vi "Init RemoteDataService.vi"(8 "error in (no error)":errorcluster, 11 "Vecto in":refnum<class "Vecto.lvclass">) -> (0 "error out":errorcluster, 3 "Vecto out":refnum<class "Vecto.lvclass">)   [LabVIEW 2020, in "Vecto.lvlib" / "Vecto.lvclass"]
uses:
  Vecto.lvclass
  Vecto.lvclass/Vecto.ctl
  RemoteDataService/RemoteDataService.lvclass
  Node Config/Node Config.lvclass
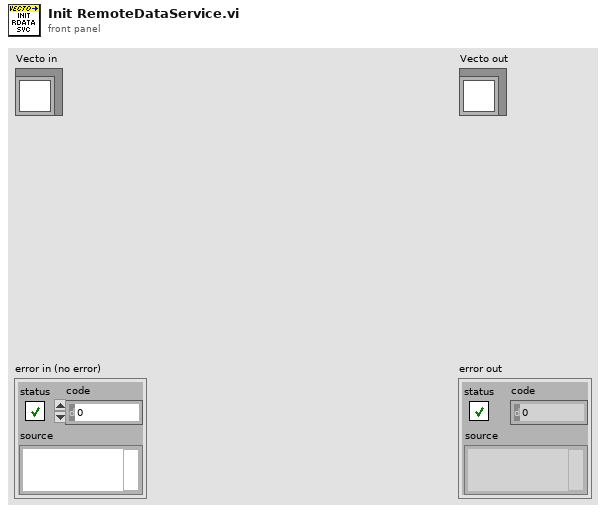
[diagram p1: front panel]
types:
  T1 = typedef "VectoConfig.lvlib/Telemetry Config.ctl" = cluster{"Routing":T2, "Endpoint":T3}
  T2 = typedef "VectoConfig.lvlib/Telemetry Routing.ctl" = enum16{"Multicast", "Unicast"}
  T3 = typedef "VectoConfig.lvlib/Endpoint.ctl" = cluster{"Address":string, "Port":u16}
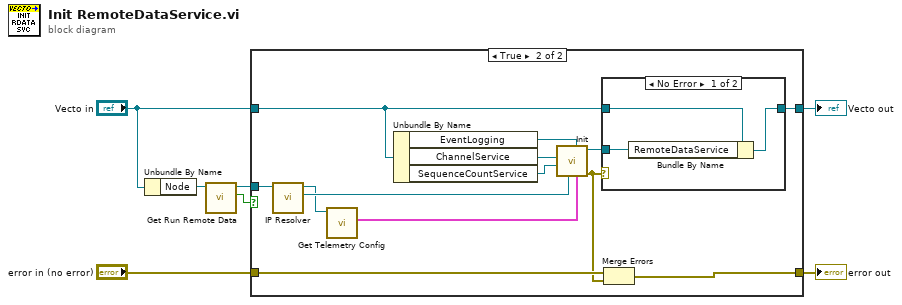
[diagram p0: block diagram]
diagram:
  n1 = Unbundle By Name("Vecto in") -> ("Node"=w5:refnum<class "Node Config.lvclass">)
  n2 = call "Get Run Remote Data.vi"("Node Config in"=w5) -> ("Run Remote Data"=w4:bool, "Node Config out"=w1:refnum<class "Node Config.lvclass">)  [unwired: 8 in, 1 out]
  n3 = case shown="True" w4 {
    tunnel: [w8 w22] -> w7
    tunnel: "Vecto in" -> [w8 w18]
    tunnel: "error in (no error)" -> [w9 w17]
    tunnel: [w9 w16] -> w2
    tunnel: w1 -> [_ w13]
    frame False {
    }
    frame True {
      n4 = call "IP Resolver.vi"("Node Config in"=w13) -> ("IP Resolver"=w12:refnum<class "IP Resolver.lvclass">, "Node Config out"=w11:refnum<class "Node Config.lvclass">)  [unwired: 8 in, 1 out]
      n5 = call "Get Telemetry Config.vi"("Node Config in"=w11) -> ("Telemtry Config"=w10:T1)  [unwired: 8 in, 2 out]
      n6 = Unbundle By Name(w18) -> ("EventLogging"=w14:refnum<class "EventLoggingService.lvclass">, "ChannelService"=w20:refnum<class "ChannelService.lvclass">, "SequenceCountService"=w19:refnum<class "SequenceCountService.lvclass">)
      n7 = call "Init.vi"("Telemtry Config (Multicast)"=w10, "EventLogger"=w14, "IP Resolver"=w12, "SequenceCountService"=w19, "ChannelService"=w20) -> ("error out"=w15:errorcluster, "RemoteDataService out"=w21:refnum<class "RemoteDataService.lvclass">)  [unwired: 5 in]
      n8 = case shown="No Error" w15 {
        tunnel: w21 -> [w25 _]
        tunnel: w18 -> [w23 w26]
        tunnel: [w24 w26] -> w22
        frame No Error {
          n9 = Bundle By Name(cluster=w23, "RemoteDataService"=w25) -> (w24:refnum<class "Vecto.lvclass">)
        }
        frame Error {
        }
      }
      n10 = Merge Errors(w17, w15) -> (w16:errorcluster)
    }
  }
  "error out" <- w2
  "Vecto out" <- w7
